vi "VarArray_Size to Same.vi"(6 "Secondary Default In":i32, 7 "Primary Default In":variant, 8 "Error In":errorcluster, 9 "Secondary Array In":i32[](array[numeric]), 10 "Select In":T1(ring), 11 "Primary Array In":variant[](array[variant])) -> (0 "Error Out":errorcluster, 1 "Secondary Array Out":i32[](array[numeric]), 3 "Primary Array Out":variant[](array[variant]))   [LabVIEW 2015]
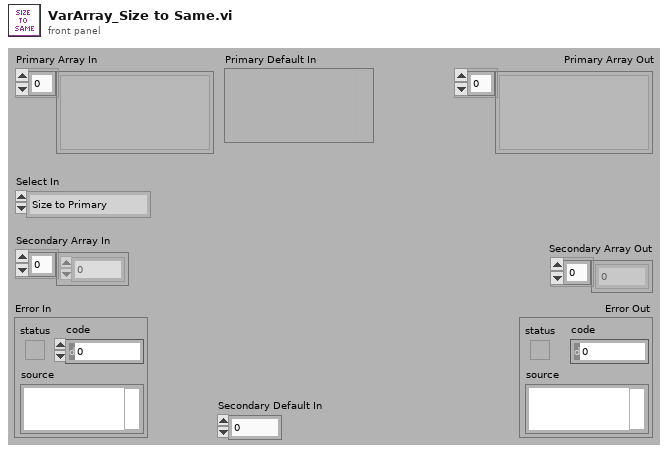
[diagram p1: front panel]
types:
  T1 = enum16{"Size to Primary", "Size to Secondary", "Size to Largest", "Size to Smallest"}
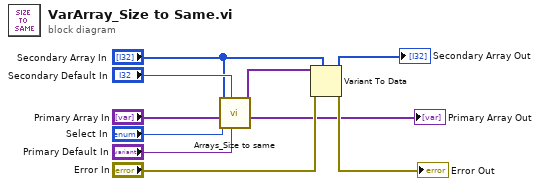
[diagram p0: block diagram]
diagram:
  n1 = call "Arrays_Size to same.vi"("Primary Default In"="Primary Default In", "Secondary Default In"="Secondary Default In", "Select In"="Select In", "Primary Array In"="Primary Array In", "Secondary Array In"="Secondary Array In") -> ("Primary Array Out"=→"Primary Array Out":variant[], "Secondary Array Out"=w4:variant[])  [unwired: 5 in]
  n2 = Variant To Data(error in="Error In", type="Secondary Array In", Variant=w4) -> (data=→"Secondary Array Out":i32[], error out=→"Error Out":errorcluster)
